vi "ToDatagram.vi"(8 "error in (no error)":errorcluster, 10 "messageID":u16, 11 "SubscribeMqttMsg in":refnum<class "SubscribeMqttMsg.lvclass">) -> (0 "error out":errorcluster, 2 "Datagram":u8[](array[numeric]), 3 "SubscribeMqttMsg out":refnum<class "SubscribeMqttMsg.lvclass">)   [LabVIEW 2020, in "SubscribeMqttMsg.lvclass"]
uses:
  SubscribeMqttMsg.lvclass
  mqttTypedef/mqttMessageType.ctl
  mqttTypedef/mqttQOSlevel.ctl
  SubscribeMqttMsg.lvclass/SubscribeMqttMsg.ctl
  MQTT Client.lvclass
  BaseMqttMsg.lvclass
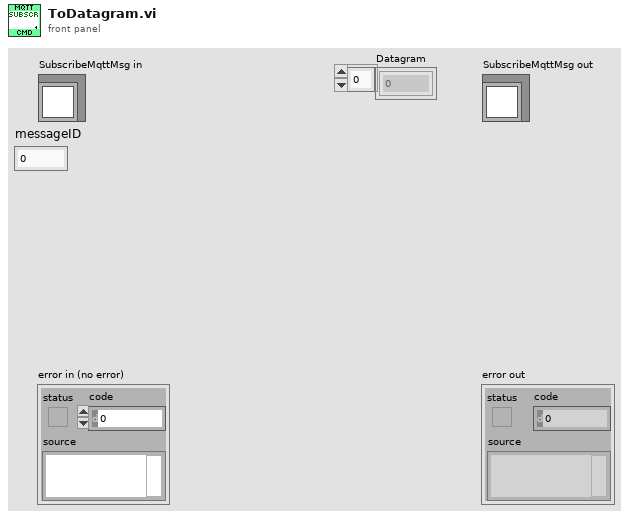
[diagram p1: front panel]
types:
  T1 = typedef "MQTT Client.lvclass/mqttQOSlevel.ctl" = enum8{"At most once", "At least once", "Exactly once", "Reserved"}
  T2 = typedef "MQTT Client.lvclass/mqttMessageType.ctl" = enum32{"Reserved", "CONNECT", "CONNACK", "PUBLISH", "PUBACK", "PUBREC", "PUBREL", "PUBCOMP", "SUBSCRIBE", "SUBACK", "UNSUBSCRIBE", "UNSUBACK", "PINGREQ", "PINGRESP", "DISCONNECT", "Reserved2"}
  T3 = typedef "MQTT Client.lvclass/mqttSubscribeCluster.ctl" = cluster{"Topic":string, "QoS":T1}
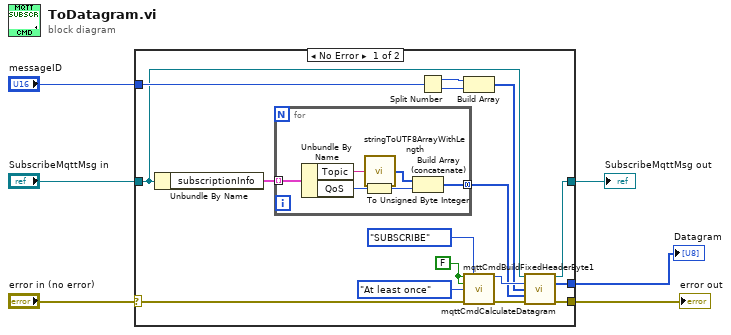
[diagram p0: block diagram]
diagram:
  n1 = case shown="No Error" "error in (no error)" {
    selector: "error in (no error)" -> [w12 w30]
    tunnel: [w8 w30] -> w5
    tunnel: [w10 w29] -> w3
    tunnel: "SubscribeMqttMsg in" -> [w13 w29]
    tunnel: "messageID" -> [w14 _]
    tunnel: [w9 _] -> w2
    frame No Error {
      w18 = FALSE ("retain(F)")
      n2 = Unbundle By Name(w13) -> ("subscriptionInfo"=w7:T3[])
      n3 = for {
        tunnel: w7 -> [w28] mode=indexing
        tunnel: [w23] -> w15 mode=concatenating
        n4 = Unbundle By Name(w28) -> ("Topic"=w27:string, "QoS"=w25:T1)
        n5 = To Unsigned Byte Integer(number=w25) -> (unsigned 8bit integer=w24:u8)
        n6 = call "stringToUTF8ArrayWithLength.vi"("string"=w27) -> ("UTF8[]"=w26:u8[])  [unwired: 14 in]
        n7 = Build Array (concatenate)(w26, w24) -> (w23:u8[])
      }
      n8 = Split Number(x=w14) -> (hi(x)=w21:u8, lo(x)=w22:u8)
      n9 = Build Array(w21, w22) -> (w16:u8[])
      n10 = call "mqttCmdBuildFixedHeaderByte1.vi"("retain(F)"=w18, "MessageType"=mqttMessageType."SUBSCRIBE", "duplicate(F)"=w18, "QoS (At most once)"=mqttQOSlevel."At least once", "error in (no error)"=w12) -> ("byte1"=w17:u8, "error out"=w11:errorcluster)  [unwired: 9 in]
      n11 = call-dynamic "mqttCmdCalculateDatagram.vi"("mqttCmd in"=w13, "FixedHeaderByte1"=w17, "variableHeader"=w16, "payload"=w15, "error in (no error)"=w11) -> ("mqttCmd out"=w10:refnum<class "SubscribeMqttMsg.lvclass">, "Datagram"=w9:u8[], "error out"=w8:errorcluster)  [unwired: 8 in]
    }
    frame Error {
    }
  }
  "error out" <- w5
  "SubscribeMqttMsg out" <- w3
  "Datagram" <- w2
